vi "G#Object_CastG#ObjectToIG#.vi"(5 "reference in":refnum<class "G#Object.lvclass">) -> (1 "not a refnum?":bool, 2 "IG# reference out":refnum<class "IG#.lvclass">)   [LabVIEW 2020, in "G#Object.lvclass"]
doc: "Cast from G#Object to the more generic IG# interface."
uses:
  <vilib>/addons/_AddQ/G#Object/G#Object.lvclass
  <vilib>/addons/_AddQ/IG#/IG#.lvclass
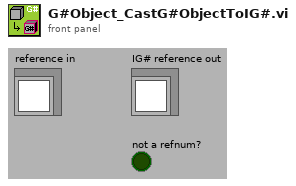
[diagram p1: front panel]
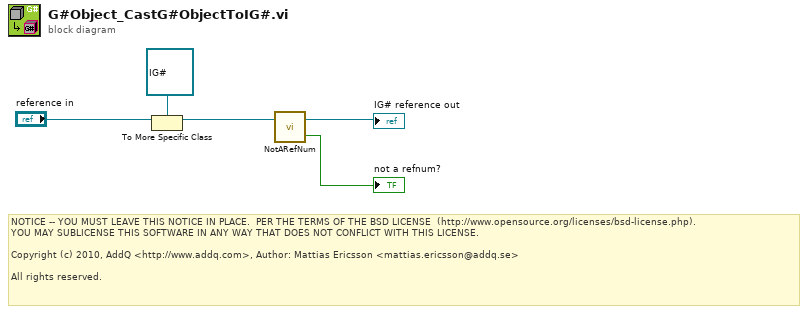
[diagram p0: block diagram]
diagram:
  # "NOTICE -- YOU MUST LEAVE THIS NOTICE IN PLACE.  PER THE TERMS OF THE BSD LICENSE  (http://www.opensource.org/licenses/bsd-license.php).\nYOU MAY SUBLICENSE THIS SOFTWARE IN ANY WAY THAT DOES NOT CONFLICT WITH THIS LICENSE.\n\nCopyright (c) 2010, AddQ <http://www.addq.com>, Author: Mattias Ericsson <mattias.ericsson@addq.se>\n\nAll rights reserved."
  n1 = To More Specific Class(target class=refnum<class "IG#.lvclass"> refnum ("IG# reference out"), reference="reference in") -> (specific class reference=w4:refnum<class "IG#.lvclass">)  [unwired: 1 in, 1 out]
  n2 = call-dynamic "NotARefNum.vi"("reference in"=w4) -> ("not a refnum?"=→"not a refnum?":bool, "reference out"=→"IG# reference out":refnum<class "IG#.lvclass">)  [unwired: 1 in]
